vi "get display name.vi"(8 "error in":errorcluster, 11 "VI modification in":refnum<class "VI modification.lvclass">) -> (0 "error out":errorcluster, 2 "class name":string, 3 "VI modification out":refnum<class "VI modification.lvclass">)   [LabVIEW 2013, in "VI modification.lvclass"]
uses:
  VI modification.lvclass
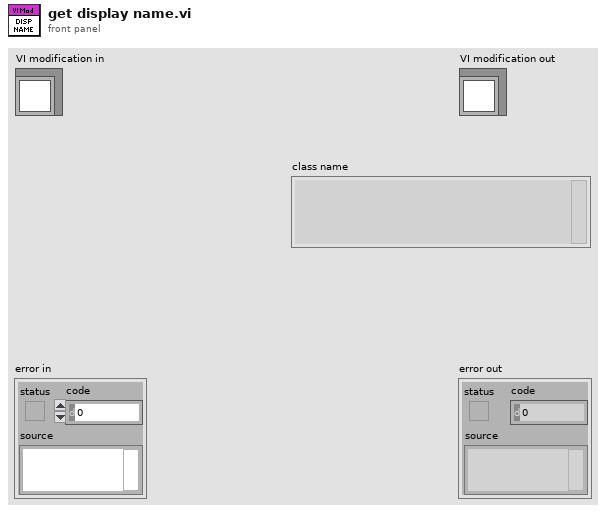
[diagram p1: front panel]
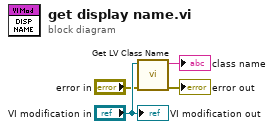
[diagram p0: block diagram]
diagram:
  n1 = call <vilib>:"Get LV Class Name.vi"("error in (no error)"="error in", "object"="VI modification in") -> ("error out"=→"error out":errorcluster, "class name"=→"class name":string)  [unwired: 8 in]
  "VI modification out" <- "VI modification in"
